vi "Main_control_cRIO.vi"() -> ()   [LabVIEW 2021]
uses:
  <vilib>/platform/TimedLoop/XDataNode/XDataNode.xnode
  <vilib>/Platform/TimedLoop/XDataNode/nitl_modes.ctl
  <vilib>/Platform/TimedLoop/XDataNode/XDNodeRunTimeDep.lvlib
  <vilib>/Platform/TimedLoop/XDataNode/wakeup.ctl
  <vilib>/Platform/TimedLoop/XDataNode/timing_clust.ctl
  <vilib>/rvi/interface/nirviOpenFPGA/nirviOpenFPGA.xnode
  <vilib>/rvi/interface/nirviReadWriteControl/nirviReadWriteControl.xnode
  <vilib>/rvi/interface/nirviCloseFPGA/nirviCloseFPGA.xnode
  SubVIs/DAQ/DAQ_Termopares.lvlib
  SubVIs/CC Modbus/CC_Library.lvlib
  <vilib>/Analysis/NI_AALBase.lvlib
  <vilib>/Analysis/baseanly.llb/Mean (DBL).vi
  <vilib>/Modbus/slave/Modbus Slave.lvclass
  a7aeaaac-04ba-4589-9d9a-9c348744fe2e.vi
  <vilib>/rvi/interface/Simulation/niFpgaSimulationCallBeginRW.vi
  <vilib>/rvi/errors/niLvFpgaAdjustHostInterfaceError.vi
  <vilib>/Modbus/master/Modbus Master.lvclass
  <vilib>/Modbus/slave/Create Slave Instance (TCP).vi
  NiFpgaLv.dll
  <vilib>/Utility/error.llb/Error Cluster From Error Code.vi
  <vilib>/FPGAPlugInAG/Dynamic/niLvFpga_Close_Dynamic.vi
  FPGA Bitfiles/pwmhybrid_FPGATarget_FPGA1_zfi6noby5Tw.lvbitx
  DEV_cRIO Bitron v9_4/FPGA_1.vi
  <vilib>/FPGAPlugInAG/cRIO-9045/niLvFpga_Open_cRIO-9045.vi
  <vilib>/rvi/interface/common/dynamic/niFpgaDynamicAddResources.vi
panel:
  in  "Activar Sim Bitron":bool
  out "LEL":bool
  out "CO":bool
  out "O2":bool
  out "LEL (%)":dbl
  out "CO (%)":dbl
  out "O2 (%)":dbl
  out "Array Warnings":bool[](array[boolean])
  out "Guardando resumen":bool=TRUE
  out "path":path
  out "T estabilidad calor":u32
  out "T transitorio calor":u32
  out "T estabilidad frio":u32
  out "T transitorio frio":u32
  out "Timer 4 (Inicio Estabilidad Calor)":u32
  out "Timer 3 (Inicio Transitorio Calor)":u32
  in  "Configuración":T1(tab)
  in  "Setpoint calor cam":dbl=55.0
  in  "Setpoints peltiers":dbl=85.0
  in  "Setpoint calor corte rampa":dbl=51.0
  in  "Setpoint Frío":dbl=-40.0 min=-28.0 max=70.0 step=0.1
  in  "Setpoint Corte Frío":dbl=-30.0 min=-28.0 max=70.0 step=0.1
  in  "Tiempò en estabilidad de Frío":u32=15
  in  "Tiempo minimo de ciclo":u32=70
  in  "Tiempo maximo de ciclo":u32=90
  in  "Cam ºC/min":dbl=2.2
  in  "Pelt ºC/min":dbl=2.5
  in  "T cliclo (Bitron FSM Sim)":u32
  in  "FSM Bitron Simulacion":i32
  out "DO H2 LAB":bool
  out "Array":dbl[][](array[numeric])
  out "error out":errorcluster
  in  "Test":bool
  in  "Disable PID":bool
  in  "Test PWM":u32[](array[numeric])
  out "PWM array":u32[](array[numeric])
  out "T_valves":dbl[](array[numeric]) format="%0.2f"
  out "PWM 8 (%)":u32
  out "PWM 7 (%)":u32
  out "PWM 6 (%)":u32
  out "PWM 5 (%)":u32
  out "PWM 4 (%)":u32
  out "PWM 3 (%)":u32=50 max=100
  out "SGL values":dbl[](array[numeric])
  out "Int values":u16[](array[numeric])
  out "Guardando en disco":bool
  out "array w/ subset deleted":dbl[][](array[numeric])
  out "Guardar Array":dbl[][](array[numeric])
  out "size(s)":i32
  out "TCP Connection Count":u32
  out "mean_T_valves":dbl format="%0.2f"
  out "Holding registers":u16[](array[numeric])
  out "First Time":bool=TRUE
  out "Timer 1 (Inicio transitorio frio)":u32
  out "Timer 2 (Inicio Estabilidad Frio)":u32
  in  "Rampa_cam":bool
  out "Temp_valves":dbl[](array[numeric]) format="%0.2f"
  in  "Rampa_pelt":bool
  in  "Minutos de medio ciclo":dbl=70.0
  out "Minutos":dbl
  out "Ciclos Totales":dbl
  out "segundos":dbl
  out "días":dbl
  out "Horas":dbl
  out "Minutos Totales":dbl
  out "t ensayo (s)":u64
  in  "Reset tempo":bool
  out "Iteration Duration":i64
  in  "Desconex_Control_Hum":bool
  out "PWM 2 (%)":u32
  out "Program running":bool
  in  "Pausa entrar":bool
  in  "Segmento":u16
  in  "Pausa":bool
  in  "stop Control General":bool
  in  "Run Program":bool
  in  "Entrada digital Bitron":bool
  in  "Cam_Hum_write":dbl min=0.0 max=100.0 step=0.1
  in  "Cam_Write_Set_Hum":bool
  in  "Cam_Temp_write":dbl min=-28.0 max=70.0 step=0.1
  in  "Cam_Write_Set_Temp":bool
  out "Cam_Temp_read":dbl min=-28.0 max=70.0 step=0.1
  out "Cam_Hum_read":dbl min=-28.0 max=70.0 step=0.1
  in  "Setpoint Peltiers":dbl=25.0
  in  "enable_PI":bool
  out "PWM 1 (%)":u32=50 max=100
  in  "STOP ALL":bool
  # "Temporizadores de ciclo"
  # "PWM1TEST"
  # "PWM2TEST"
  # "PWM3TEST"
  # "PWM4TEST"
  # "PWM5TEST"
  # "PWM6TEST"
  # "PWM7TEST"
  # "PWM8TEST"
  # "Peltier_1"
  # "Cámara climática"
  # "min"
  # "min"
  # "min"
  # "min"
  # "segmento"
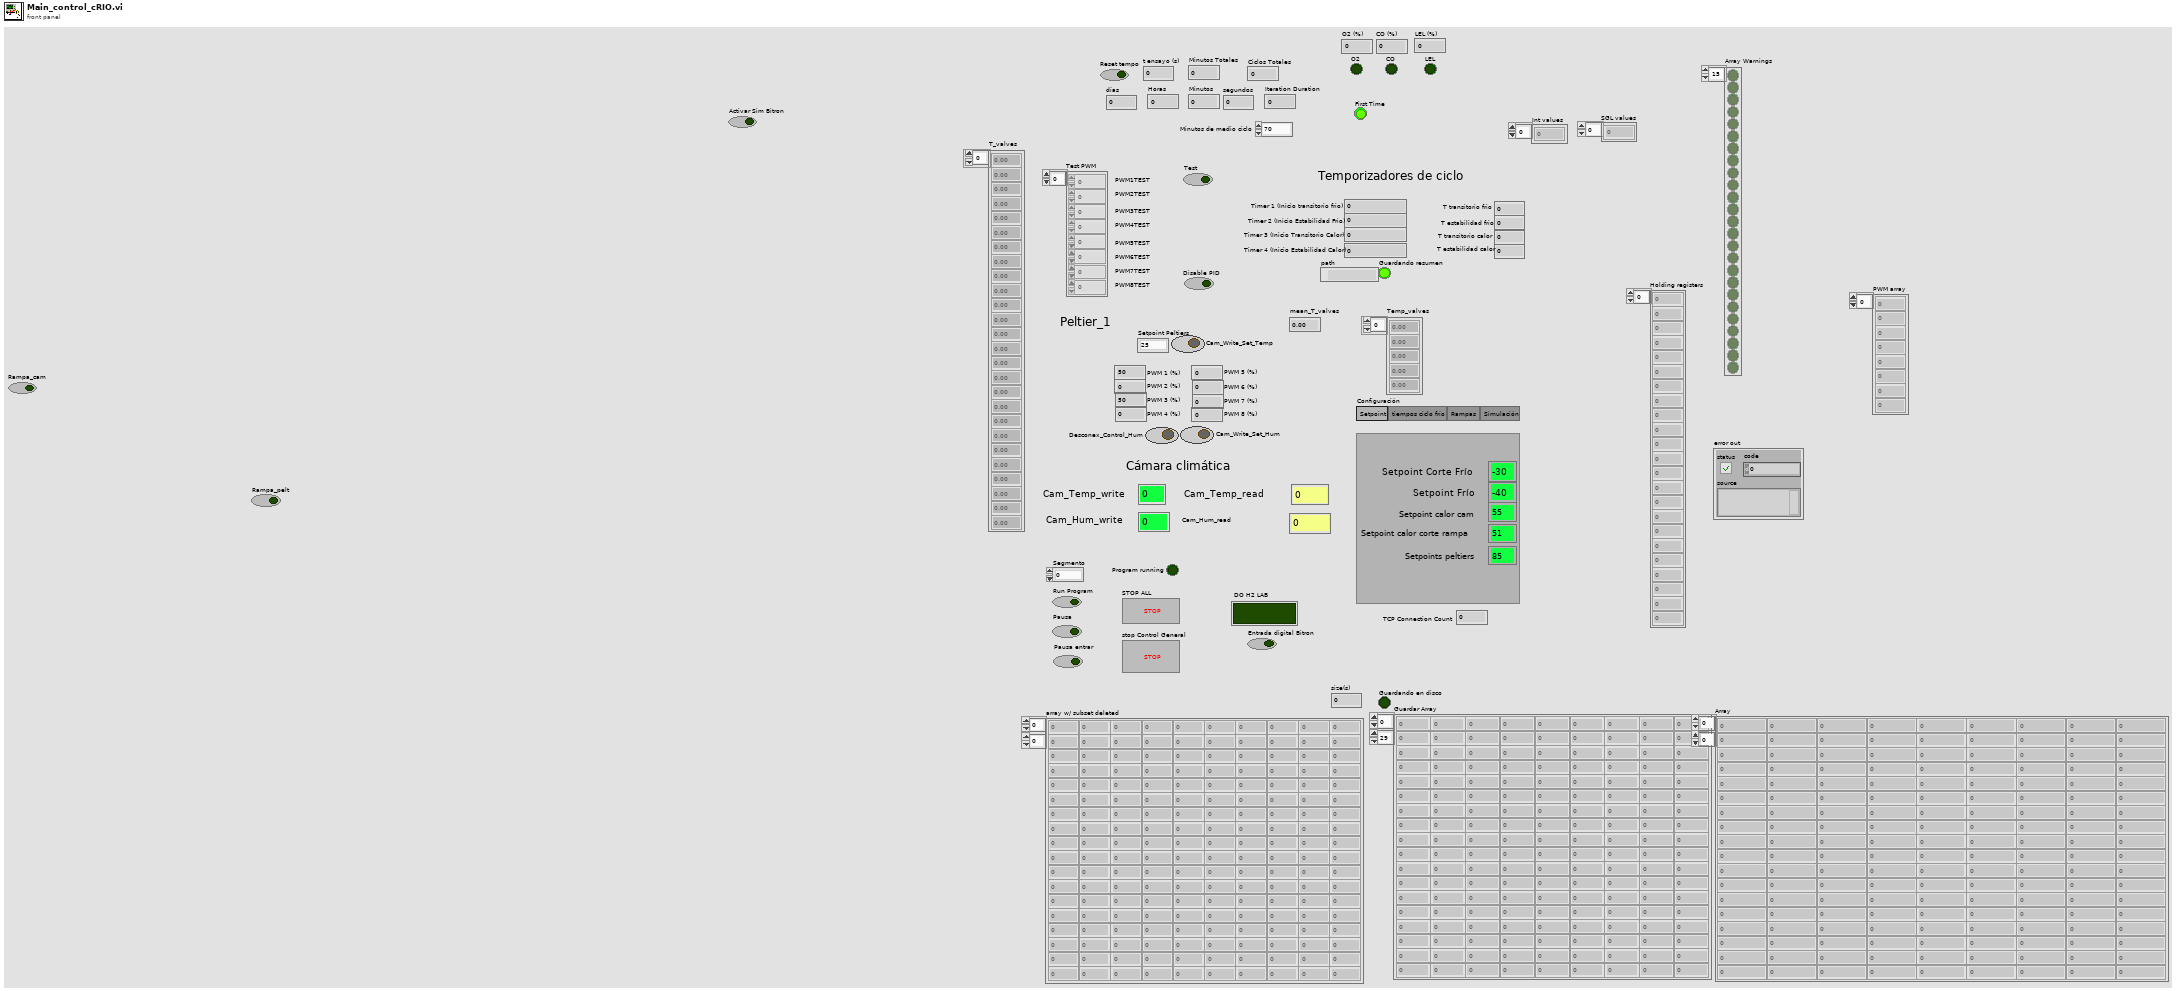
[diagram p1: front panel]
types:
  T1 = enum32{"Setpoint", "tiempos ciclo frío", "Rampas ", "Simulación"}
  T2 = enum8{"Enabled", "Disabled", "Disabled and Grayed Out"}
  T3 = typedef "XDNodeRunTimeDep.lvlib/timing_clust.ctl" = cluster{"Expected End [f-1]":u64, "Actual End [f-1]":u64, "Finished Late? [f-1]":bool, "Expected End [i-1]":u64, "Actual End [i-1]":u64, "Finished Late? [i-1]":bool, "Expected Start [i]":u64, "Actual Start [i]":u64, "Expected Start [f]":u64, "Actual Start [f]":u64, "Source Name":string, "Structure Name":string, "Period":i64, "Deadline":i64, "Offset":i64, "Start":i64, "Priority":i32, "Timeout":i32, "Mode":T4, "Wakeup Reason":T5, "Error":errorcluster, "Source Type":string, "Secondary Source Type":string, "Global End Time":u64, "Global Start Time":u64, "Frame Duration":u64, "Iteration Duration":u64, "Assigned CPU":i32, "I/O Scan Engine Mode":u32}
  T4 = typedef "XDNodeRunTimeDep.lvlib/nitl_modes.ctl" = enum32{"No Change", "Process missed periods, maintain original phase", "Discard missed periods, maintain original phase", "Process missed periods, ignore original phase", "Discard missed periods, ignore original phase"}
  T5 = typedef "XDNodeRunTimeDep.lvlib/wakeup.ctl" = enum32{"Normal", "Aborted", "Asynchronous wakeup", "Timing source error", "Timed loop error", "Timeout"}
  T6 = enum16{"open", "open or create", "create or replace", "create", "open (read-only)"}
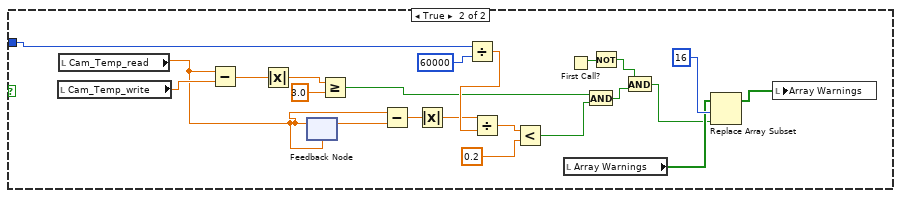
[diagram p3: hidden frame]
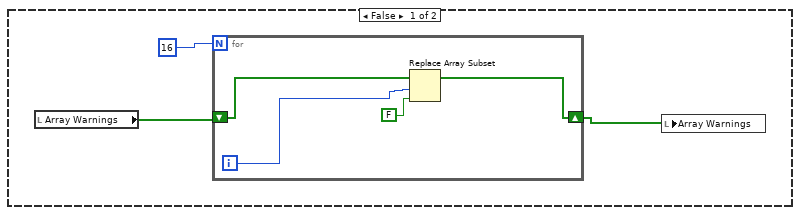
[diagram p4: hidden frame]
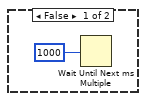
[diagram p7: hidden frame]
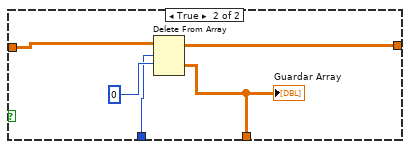
[diagram p8: hidden frame]
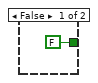
[diagram p9: hidden frame]
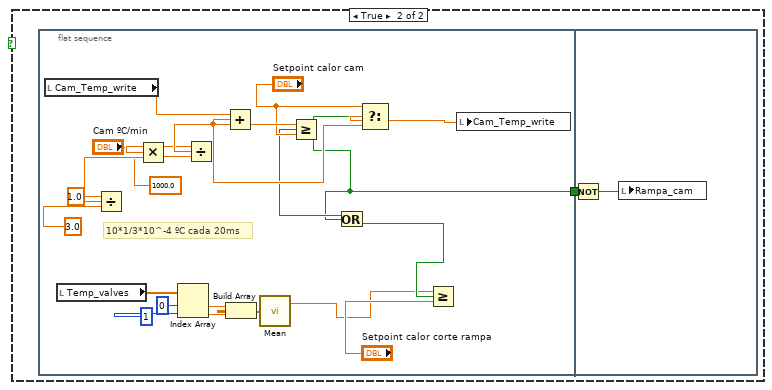
[diagram p12: hidden frame]
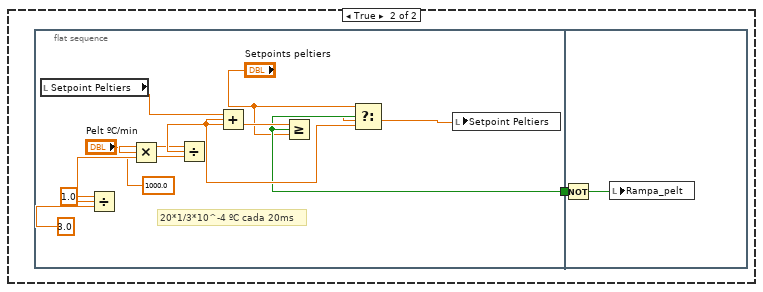
[diagram p13: hidden frame]
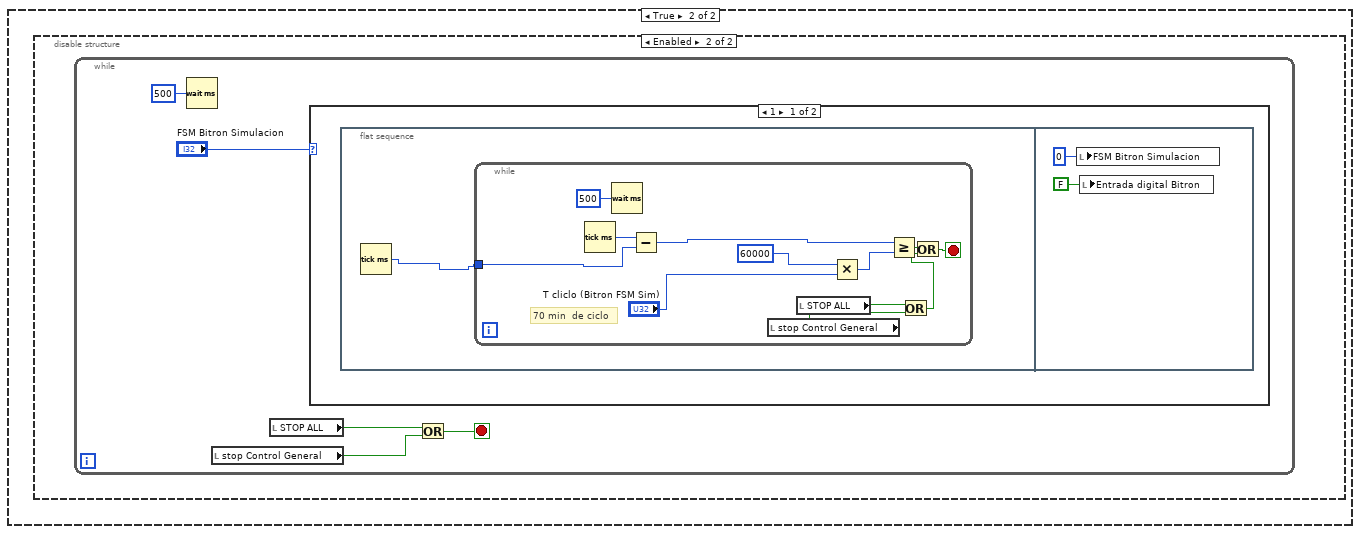
[diagram p14: hidden frame]
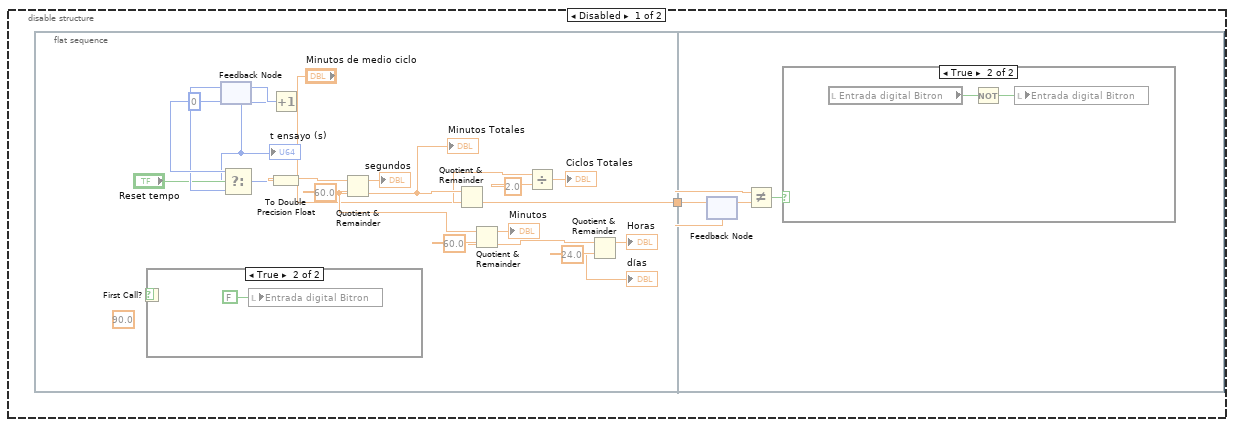
[diagram p15: hidden frame]
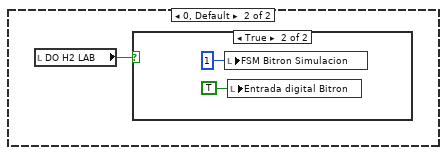
[diagram p18: hidden frame]
diagram:
  n1 = flat-sequence {
    tunnel: [w25] -> w15
    tunnel: [w24] -> w12
    tunnel: [w20] -> w11
    tunnel: [w27] -> w8
    tunnel: [w26] -> w7
    tunnel: [w17] -> w4
    tunnel: [w16] -> w3
    tunnel: w15 -> [w58]
    tunnel: [w57] -> w14
    tunnel: [w56] -> w13
    tunnel: w12 -> [w55]
    tunnel: w11 -> [_]
    tunnel: [w48] -> w10
    tunnel: [w47] -> w9
    tunnel: w8 -> [w44]
    tunnel: w7 -> [w43]
    tunnel: [w42] -> w6
    tunnel: [w41] -> w5
    tunnel: w4 -> [_]
    tunnel: w3 -> [_]
    tunnel: [w29] -> w2
    tunnel: [w30] -> w1
    tunnel: w14 -> [w815]
    tunnel: w13 -> [w814]
    tunnel: w10 -> [w823]
    tunnel: w9 -> [w822]
    tunnel: w6 -> [w818]
    tunnel: w5 -> [w817]
    tunnel: w2 -> [w809]
    tunnel: w1 -> [w810]
    frame #0 {
      w16 = bool[] [FALSE, FALSE, FALSE, FALSE, FALSE, FALSE, FALSE, FALSE, FALSE, FALSE, FALSE, FALSE, FALSE, FALSE, FALSE, FALSE, FALSE, FALSE, FALSE] ("Array Warnings")
      w17 = FALSE ("DO H2 LAB")
      w18 = u32 0 ("PWM 1 (%)")
      w22 = TRUE ("Visible")
      w28 = 10086 items=["J"=10072, "K"=10073, "N"=10077, "R"=10082, "S"=10085, "T"=10086, "B"=10047, "E"=10055] ("thermocouple type")
      w20 = FALSE ("Visible")
      n2 = local write "Entrada digital Bitron"(FALSE ("Entrada digital Bitron")) -> ()
      n3 = call "DAQ_connect.vi"("thermocouple type"=w28, "Array"=tag[] ["Mod2/ai0", "Mod2/ai1", "Mod2/ai2", "Mod2/ai3", "Mod2/ai4", "Mod2/ai5", "Mod2/ai6", "Mod2/ai7", "Mod2/ai8", "Mod2/ai9", "Mod2/ai10", "Mod2/ai11", "Mod2/ai12", "Mod2/ai13", "Mod2/ai14", "Mod2/ai15"]) -> ("error out"=w26:errorcluster, "Refnum out"=w27:refnum<k21>)  [unwired: 8 in]
      "error out" <- w26
      n4 = property on="Cam_Write_Set_Temp" class="Bool (strict)"("Visible"=w22) -> ()  [unwired: 2 in, 2 out]
      n5 = local write "PWM 8 (%)"(w18) -> ()
      n6 = property on="Cam_Write_Set_Hum" class="Bool (strict)"("Visible"=w22) -> ()  [unwired: 2 in, 2 out]
      n7 = local write "PWM 6 (%)"(w18) -> ()
      n8 = local write "PWM 7 (%)"(w18) -> ()
      n9 = local write "PWM 5 (%)"(w18) -> ()
      n10 = local write "PWM 4 (%)"(w18) -> ()
      n11 = local write "PWM 1 (%)"(w18) -> ()
      n12 = local write "PWM 2 (%)"(w18) -> ()
      n13 = local write "Rampa_pelt"(w20) -> ()
      n14 = local write "PWM 3 (%)"(w18) -> ()
      n15 = property on="enable_PI" class="Bool (strict)"("Visible"=w20) -> ()  [unwired: 2 in, 2 out]
      n16 = xnode "Open FPGA VI Reference"() -> ("FPGA VI Reference Out"=w25:refnum<k20>, "error out"=w24:errorcluster)  [unwired: 2 in]
      n17 = property on="Disable PID" class="Bool (strict)"("DisabledEnum"=T2."Disabled" ("Disabled")) -> ()  [unwired: 2 in, 2 out]
      "DO H2 LAB" <- w17
      "Array Warnings" <- w16
    }
    frame #1 {
      # "Running"
      n18 = node-c288() -> (w36:T3)  [unwired: 4 in]
      n19 = node-c288() -> (w60:T3)  [unwired: 4 in]
      n20 = node-c288() -> (w34:T3)  [unwired: 4 in]
      n21 = call "Nanodac_connect.vi"() -> ("error out"=w31:errorcluster, "Modbus Master out"=w32:refnum<class "Modbus Master.lvclass">)  [unwired: 10 in]
      n22 = while "Adquisicion Resumen Datos/ciclo" {
        stop <- w170 stop-if-true
        w171 = FALSE ("Guardando resumen")
        # "CUIDADO! Al volver a empezar el ciclo, el Timer 1 va a ser el del siguiente ciclo, no el del que queremos registrar"
        # "0 -> First Time. Frío hasta -30 y señal bitron\n1 -> Transitorio frio\n2 -> Estabilidad frio\n3 -> Transitorio calor\n4 -> Estabilidad calor"
        # "Datos a guardar por ciclo:\n- Tiempo semiciclo frio\n- Tiempo estabilidad frio\n- Tiempo semiciclo calor\n- Tiempo estabilidad calor"
        n23 = local read "Segmento"() -> (w182:u16)
        n24 = feedback-in #1(w182) -> ()
        n25 = feedback #1(w182) -> (w181:u16)
        n26 = Equal?(x=w182, y=u16 1) -> (x = y?=w179:bool)
        n27 = local read "Program running"() -> (w168:bool)
        n28 = local write "Guardando resumen"(w171) -> ()
        n29 = local read "Segmento"() -> (w173:u16)
        n30 = Not Equal?(x=w181, y=u16 1) -> (x != y?=w178:bool)
        n31 = And(x=w179, y=w178) -> (x .and. y?=w169:bool)
        n32 = And(x=w168, y=w169) -> (x .and. y?=w167:bool)
        n33 = feedback #2(w173) -> (w174:u16)
        n34 = feedback-in #2(w173) -> ()
        n35 = Equal?(x=w173, y=u16 4) -> (x = y?=w176:bool)
        n36 = local read "Program running"() -> (w164:bool)
        n37 = case shown="True" w167 {
          tunnel: w171 -> [_ _]
          frame False {
          }
          frame True {
            n38 = flat-sequence {
              frame #0 {
                n39 = local read "Timer 4 (Inicio Estabilidad Calor)"() -> (w188:u32)
                n40 = local read "Timer 3 (Inicio Transitorio Calor)"() -> (w190:u32)
                n41 = local read "Timer 2 (Inicio Estabilidad Frio)"() -> (w191:u32)
                n42 = local read "Timer 1 (Inicio transitorio frio)"() -> (w189:u32)
                n43 = Subtract(x=w189, y=w188) -> (x-y=→"T estabilidad calor":u32)
                n44 = Subtract(x=w188, y=w190) -> (x-y=→"T transitorio calor":u32)
                n45 = Subtract(x=w190, y=w191) -> (x-y=→"T estabilidad frio":u32)
              }
              frame #1 {
                n46 = while {
                  stop <- w195 stop-if-true
                  n47 = local read "Guardando en disco"() -> (w196:bool)
                  n48 = Not(x=w196) -> (.not. x?=w195:bool)
                  n49 = Wait (ms)(milliseconds to wait=u32 500) -> ()  [unwired: 1 out]
                }
              }
              frame #2 {
                n50 = local read "T estabilidad frio"() -> (w203:u32)
                n51 = local read "T transitorio calor"() -> (w202:u32)
                n52 = local read "path"() -> (w199:path)
                n53 = local read "T transitorio frio"() -> (w204:u32)
                n54 = local read "T estabilidad calor"() -> (w201:u32)
                n55 = TDMS Open(10:T6."open or create" ("operation (0:open)"), 11:w199) -> (0:w209:errorcluster, 3:w210:refnum<k34>)  [unwired: 5 in]
                n56 = Build Array(w204, w203, w202, w201) -> (w200:u32[])
                n57 = TDMS Write(0:w210, 5:"Resumen Ciclos" ("group name in (Untitled)"), 7:string[] ["Time Transitorio frio (s)", "Time estabilidad frio (s)", "Time Transitorio calor (s)", "Time estabilidad calor (s)"] ("channel name(s) in (Untitled)"), 9:w200, 11:w209) -> (4:w208:refnum<k34>, 15:w207:errorcluster)  [unwired: 1 in, 2 out]
                n58 = TDMS Close(8:w207, 11:w208) -> ()  [unwired: 2 out]
                "Guardando resumen" <- TRUE
              }
            }
          }
        }
        n59 = Not Equal?(x=w174, y=u16 4) -> (x != y?=w177:bool)
        n60 = And(x=w176, y=w177) -> (x .and. y?=w166:bool)
        n61 = And(x=w166, y=w164) -> (x .and. y?=w165:bool)
        n62 = case shown="True" w165 {
          frame False {
          }
          frame True {
            n63 = local read "Timer 1 (Inicio transitorio frio)"() -> (w185:u32)
            n64 = local read "Timer 2 (Inicio Estabilidad Frio)"() -> (w184:u32)
            n65 = Subtract(x=w184, y=w185) -> (x-y=→"T transitorio frio":u32)
          }
        }
        n66 = local read "STOP ALL"() -> (w170:bool)
        n67 = Wait (ms)(milliseconds to wait=u32 500) -> ()  [unwired: 1 out]
      }
      n68 = timed-loop "Rampa SP Camara" {
        timing: w36 -> [_]
        timing-out: [_] -> w35
        stop <- w435 stop-if-true
        n69 = node-c288() -> ()  [unwired: 1 in, 1 out]
        n70 = case shown="False" "Rampa_cam" {
          frame False {
            n71 = Wait (ms)(milliseconds to wait=u32 500) -> ()  [unwired: 1 out]
          }
          frame True {
            n72 = flat-sequence {
              tunnel: [w445] -> w437
              tunnel: w437 -> [w460]
              frame #0 {
                # "10*1/3*10^-4 ºC cada 20ms"
                n73 = local read "Cam_Temp_write"() -> (w451:dbl)
                n74 = local read "Temp_valves"() -> (w443:dbl[])
                n75 = Divide(x=1.0, y=3.0) -> (x/y=w457:dbl)
                n76 = Multiply(x="Cam ºC/min", y=w457) -> (x*y=w455:dbl)
                n77 = Index Array(array=w443, index #1=0 ("index"), index #2=1 ("index")) -> (element #1=w440:dbl, element #2=w439:dbl)
                n78 = Divide(x=w455, y=1000.0) -> (x/y=w456:dbl)
                n79 = Add(x=w451, y=w456) -> (x+y=w453:dbl)
                n80 = Build Array(w440, w439) -> (w438:dbl[])
                n81 = call-poly <vilib>:"Mean.vi"("X"=w438) -> ("mean"=w444:dbl)  [unwired: 1 out]
                n82 = Greater Or Equal?(x=w453, y="Setpoint calor cam") -> (x >= y?=w446:bool)
                n83 = Greater Or Equal?(x=w444, y="Setpoint calor corte rampa") -> (x >= y?=w447:bool)
                n84 = Or(x=w446, y=w447) -> (x .or. y?=w445:bool)
                n85 = Select(t="Setpoint calor cam", s=w445, f=w453) -> (s? t:f=w452:dbl)
                n86 = local write "Cam_Temp_write"(w452) -> ()
              }
              frame #1 {
                n87 = Not(x=w460) -> (.not. x?=w461:bool)
                n88 = local write "Rampa_cam"(w461) -> ()
              }
            }
          }
        }
        n89 = local read "STOP ALL"() -> (w435:bool)
        n90 = node-c288() -> ()  [unwired: 1 in, 1 out]
      }
      n91 = timed-loop "FPGA Aquisicion y control" {
        timing: w60 -> [_]
        timing-out: [_] -> w59
        tunnel: w58 -> [w802]
        tunnel: [w801] -> w57
        tunnel: [w800] -> w56
        tunnel: w55 -> [w799]
        tunnel: w44 -> [w798]
        tunnel: w43 -> [w797]
        tunnel: [w796] -> w42
        tunnel: [w795] -> w41
        stop <- "STOP ALL" stop-if-true
        # "1 y 1 de momento, cuando haya mas valvulas, 2 y 2"
        n92 = node-c288() -> ()  [unwired: 1 in, 1 out]
        n93 = local read "PWM 8 (%)"() -> (w779:u32)
        n94 = local read "PWM 6 (%)"() -> (w781:u32)
        n95 = local read "PWM 7 (%)"() -> (w780:u32)
        n96 = local read "PWM 5 (%)"() -> (w782:u32)
        n97 = local read "PWM 4 (%)"() -> (w783:u32)
        n98 = local read "PWM 1 (%)"() -> (w786:u32)
        n99 = local read "PWM 2 (%)"() -> (w785:u32)
        n100 = local read "PWM 3 (%)"() -> (w784:u32)
        n101 = xnode "Read/Write Control"("FPGA VI Reference In"=w802, "error in"=w799) -> ("FPGA VI Reference Out"=w801:refnum<k20>, "error out"=w800:errorcluster)  [unwired: 8 in]
        n102 = call "DAQ_read_T_dT.vi"("error in (no error)"=w797, "Refnum in"=w798) -> ("error out"=w795:errorcluster, "data"=w794:dbl[], "Refnum out"=w796:refnum<k21>)  [unwired: 7 in]
        "Temp_valves" <- w794
        "T_valves" <- w794
        n103 = Build Array(w786, w785, w784, w783, w782, w781, w780, w779) -> (→"PWM array":u32[])
        n104 = call "Sort 1D Array.vim"("unsorted array"=w794) -> ("sorted array"=w790:dbl[])  [unwired: 10 in]
        n105 = Array Size(array=w790) -> (size(s)=w792:i32)
        n106 = Subtract(x=w792, y=1) -> (x-y=w793:i32)
        n107 = Array Subset(array=w790, index=1, length=w793) -> (w788:dbl[])
        n108 = call-poly <vilib>:"Mean.vi"("X"=w788) -> ("mean"=→"mean_T_valves":dbl)  [unwired: 1 out]
        n109 = node-c288() -> ()  [unwired: 1 in, 1 out]
      }
      n110 = timed-loop "Warnings/Errores" {
        timing: w34 -> [_]
        timing-out: [_] -> w33
        stop <- w74 stop-if-true
        n111 = node-c288() -> ()  [unwired: 1 in, 1 out]
        n112 = local read "Program running"() -> (w77:bool)
        n113 = local read "Pausa"() -> (w78:bool)
        n114 = Not(x=w78) -> (.not. x?=w76:bool)
        n115 = And(x=w77, y=w76) -> (x .and. y?=w75:bool)
        n116 = case shown="True" w75 {
          frame False {
          }
          frame True {
            # "0 -> First Time. Frío hasta -30 y señal bitron\n1 -> Transitorio frio\n2 -> Estabilidad frio\n3 -> Transitorio calor\n4 -> Estabilidad calor"
            # "Si estamos en semiciclo de calor\ny no hay pausa"
            n117 = local read "Segmento"() -> (w110:u16)
            n118 = Tick Count (ms)() -> (millisecond timer value=w104:u32)
            n119 = local read "LEL (%)"() -> (w96:dbl)
            n120 = feedback-in #3(w104) -> ()
            n121 = feedback #3(w104) -> (w103:u32)
            n122 = local read "Array Warnings"() -> (w92:bool[])
            n123 = Equal?(x=w110, y=u16 3) -> (x = y?=w107:bool)
            n124 = Equal?(x=w110, y=u16 4) -> (x = y?=w106:bool)
            n125 = Subtract(x=w104, y=w103) -> (x-y=w101:u32)
            n126 = Greater?(x=w96, y=3.0) -> (0:w90:bool)
            n127 = Or(x=w107, y=w106) -> (x .or. y?=w105:bool)
            n128 = Replace Array Subset(array=w92, new element=w90, index=17) -> (w89:bool[])
            n129 = Greater Or Equal?(x=w101, y=u32 1000) -> (x >= y?=w100:bool)
            n130 = Array Subset(array=w89, index=0, length=19) -> (w82:bool[])
            n131 = case shown="True" w105 {
              frame False {
                n132 = local read "Array Warnings"() -> (w138:bool[])
                n133 = for {
                  N: 16 -> [_]
                  shift-right: [w140] -> w137
                  shift-left: w138 -> [w141]
                  i -> [w143]
                  n134 = Replace Array Subset(array=w141, new element=FALSE ("new element/subarray"), index=w143) -> (w140:bool[])
                }
                n135 = local write "Array Warnings"(w137) -> ()
              }
              frame True {
                n136 = local read "Array Warnings"() -> (w145:bool[])
                n137 = local read "Setpoint Peltiers"() -> (w148:dbl)
                n138 = local read "T_valves"() -> (w147:dbl[])
                n139 = for {
                  N: 16 -> [_]
                  tunnel: w148 -> [w155]
                  tunnel: w147 -> [w153]
                  shift-right: [w149] -> w144
                  shift-left: w145 -> [w150]
                  i -> [w152]
                  n140 = Index Array(array=w153, index=w152) -> (element=w151:dbl)
                  n141 = Subtract(x=w155, y=w151) -> (x-y=w158:dbl)
                  n142 = Absolute Value(x=w158) -> (abs(x)=w157:dbl)
                  n143 = Greater?(x=w157, y=20.0) -> (0:w154:bool)
                  n144 = Replace Array Subset(array=w150, new element=w154, index=w152) -> (w149:bool[])
                }
                n145 = local write "Array Warnings"(w144) -> ()
              }
            }
            n146 = case shown="False" w100 {
              tunnel: w101 -> [_ w132]
              frame False {
                n147 = local read "Array Warnings"() -> (w114:bool[])
                n148 = Replace Array Subset(array=w114, new element=FALSE ("new element/subarray"), index=16) -> (w111:bool[])
                n149 = local write "Array Warnings"(w111) -> ()
              }
              frame True {
                n150 = local read "Cam_Temp_write"() -> (w121:dbl)
                n151 = local read "Cam_Temp_read"() -> (w119:dbl)
                n152 = Subtract(x=w119, y=w121) -> (x-y=w136:dbl)
                n153 = Absolute Value(x=w136) -> (abs(x)=w135:dbl)
                n154 = feedback #4(w119) -> (w120:dbl)
                n155 = feedback-in #4(w119) -> ()
                n156 = Greater Or Equal?(x=w135, y=3.0) -> (x >= y?=w126:bool)
                n157 = Subtract(x=w119, y=w120) -> (x-y=w133:dbl)
                n158 = Absolute Value(x=w133) -> (abs(x)=w129:dbl)
                n159 = Divide(x=w132, y=u32 60000) -> (x/y=w130:dbl)
                n160 = Divide(x=w129, y=w130) -> (x/y=w128:dbl)
                n161 = Less?(x=w128, y=0.2) -> (x < y?=w125:bool)
                n162 = local read "Array Warnings"() -> (w116:bool[])
                n163 = First Call?() -> (First Call?: T/F=w122:bool)
                n164 = And(x=w126, y=w125) -> (x .and. y?=w124:bool)
                n165 = Not(x=w122) -> (.not. x?=w123:bool)
                n166 = And(x=w123, y=w124) -> (x .and. y?=w115:bool)
                n167 = Replace Array Subset(array=w116, new element=w115, index=16) -> (w118:bool[])
                n168 = local write "Array Warnings"(w118) -> ()
              }
            }
            n169 = local write "Array Warnings"(w82) -> ()
            n170 = local read "O2 (%)"() -> (w81:dbl)
            n171 = local read "Array Warnings"() -> (w95:bool[])
            n172 = Greater?(x=w81, y=25.0) -> (0:w97:bool)
            n173 = Less?(x=w81, y=10.0) -> (x < y?=w79:bool)
            n174 = Or(x=w97, y=w79) -> (x .or. y?=w93:bool)
            n175 = Replace Array Subset(array=w95, new element=w93, index=18) -> (w84:bool[])
            n176 = Array Subset(array=w84, index=0, length=19) -> (w83:bool[])
            n177 = local write "Array Warnings"(w83) -> ()
          }
        }
        n178 = local read "STOP ALL"() -> (w74:bool)
        n179 = node-c288() -> ()  [unwired: 1 in, 1 out]
      }
      n180 = while "MODBUS CC NANODAC" {
        tunnel: w32 -> [w73]
        tunnel: w31 -> [w72]
        tunnel: [w62] -> w30
        tunnel: [w61] -> w29
        stop <- w71 stop-if-true
        n181 = call "Nanodac_lectura.vi"("Modbus Master in"=w73, "error in (no error)"=w72) -> ("Modbus Master out"=w62:refnum<class "Modbus Master.lvclass">, 16:"O2, CO, LEL"=w69:dbl[], 17:"O2, CO, LEL"=w70:bool[], "error out"=w61:errorcluster)  [unwired: 14 in]
        n182 = Index Array(array=w70) -> (element #1=→"O2":bool, element #2=→"CO":bool, element #3=→"LEL":bool)  [unwired: 3 in]
        n183 = Index Array(array=w69) -> (element #1=→"O2 (%)":dbl, element #2=→"CO (%)":dbl, element #3=→"LEL (%)":dbl)  [unwired: 3 in]
        n184 = local read "STOP ALL"() -> (w71:bool)
      }
      n185 = node-c288(w35) -> ()  [unwired: 1 out]
      n186 = node-c288() -> (w38:T3)  [unwired: 4 in]
      n187 = timed-loop "Rampa SP Peltiers" {
        timing: w38 -> [_]
        timing-out: [_] -> w37
        stop <- w467 stop-if-true
        n188 = node-c288() -> ()  [unwired: 1 in, 1 out]
        n189 = case shown="False" "Rampa_pelt" {
          frame False {
            n190 = Wait (ms)(milliseconds to wait=u32 500) -> ()  [unwired: 1 out]
          }
          frame True {
            n191 = flat-sequence {
              tunnel: [w474] -> w469
              tunnel: w469 -> [w482]
              frame #0 {
                # "20*1/3*10^-4 ºC cada 20ms"
                n192 = local read "Setpoint Peltiers"() -> (w472:dbl)
                n193 = Divide(x=1.0, y=3.0) -> (x/y=w479:dbl)
                n194 = Multiply(x="Pelt ºC/min", y=w479) -> (x*y=w477:dbl)
                n195 = Divide(x=w477, y=1000.0) -> (x/y=w478:dbl)
                n196 = Add(x=w472, y=w478) -> (x+y=w475:dbl)
                n197 = Greater Or Equal?(x=w475, y="Setpoints peltiers") -> (x >= y?=w474:bool)
                n198 = Select(t="Setpoints peltiers", s=w474, f=w475) -> (s? t:f=w473:dbl)
                n199 = local write "Setpoint Peltiers"(w473) -> ()
              }
              frame #1 {
                n200 = Not(x=w482) -> (.not. x?=w483:bool)
                n201 = local write "Rampa_pelt"(w483) -> ()
              }
            }
          }
        }
        n202 = local read "STOP ALL"() -> (w467:bool)
        n203 = node-c288() -> ()  [unwired: 1 in, 1 out]
      }
      n204 = node-c288(w59) -> ()  [unwired: 1 out]
      n205 = while "Guardado de Datos" {
        stop <- w212 stop-if-true
        n206 = local read "Program running"() -> (w211:bool)
        n207 = case shown="True" w211 {
          frame False {
            n208 = Wait Until Next ms Multiple(millisecond multiple=u32 1000 ("milliseconds to wait")) -> ()  [unwired: 1 out]
          }
          frame True {
            w222 = dbl[][] []
            n209 = Get Date/Time In Seconds() -> (seconds since 1Jan1904=w221:timestamp)
            n210 = Format Date/Time String(time format string (%c)="%Y_%m_%d_%H_%M", seconds (now)=w221) -> (date/time string=w217:string)  [unwired: 1 in]
            n211 = local write "array w/ subset deleted"(w222) -> ()
            n212 = local write "Guardar Array"(w222) -> ()
            n213 = Concatenate Strings("/media/sdb1/Datos_Bitron/" ("string"), w217, "_data CC.tdms" ("string")) -> (w218:string)
            n214 = String To Path(string=w218) -> (path=w215:path)
            "path" <- w215
            n215 = while {
              shift-right: [w272] -> _
              shift-left: w222 -> [w275]
              tunnel: w215 -> [w263]
              tunnel: [FALSE ("stop Control General")] -> w214
              i -> [w280]
              stop <- w246 stop-if-true
              # "10 minutos = 599"
              n216 = local read "Program running"() -> (w240:bool)
              n217 = local read "enable_PI"() -> (w239:bool)
              n218 = local read "Entrada digital Bitron"() -> (w238:bool)
              n219 = local read "Run Program"() -> (w237:bool)
              n220 = local read "Pausa"() -> (w236:bool)
              n221 = local read "Pausa entrar"() -> (w235:bool)
              n222 = local read "stop Control General"() -> (w234:bool)
              n223 = local read "DO H2 LAB"() -> (w231:bool)
              n224 = local read "TCP Connection Count"() -> (w252:u32)
              n225 = local read "SGL values"() -> (w261:dbl[])
              n226 = local read "Int values"() -> (w262:u16[])
              n227 = local read "Array Warnings"() -> (w225:bool[])
              n228 = Tick Count (ms)() -> (millisecond timer value=w266:u32)
              n229 = To Double Precision Float(number=w262) -> (double precision float=w260:dbl[])
              n230 = To Double Precision Float(number=w261) -> (double precision float=w259:dbl[])
              n231 = Divide(x=w266, y=u32 1000) -> (x/y=w258:dbl)
              n232 = Greater?(x=w252, y=u32 0) -> (0:w250:bool)
              n233 = Boolean To (0,1)(Boolean=w250) -> (0, 1=w254:i16)
              n234 = To Double Precision Float(number=w254) -> (double precision float=w253:dbl)
              n235 = Build Array(w240, w239, w238, w237, w236, w235, w234, w231) -> (w233:bool[])
              n236 = Boolean To (0,1)(Boolean=w225) -> (0, 1=w226:i16[])
              n237 = Build Array(w253) -> (w232:dbl[])
              n238 = Boolean To (0,1)(Boolean=w233) -> (0, 1=w256:i16[])
              n239 = To Double Precision Float(number=w226) -> (double precision float=w224:dbl[])
              n240 = Build Array(w258) -> (w257:dbl[])
              n241 = To Double Precision Float(number=w256) -> (double precision float=w255:dbl[])
              n242 = Transpose 2D Array(2D array=w275) -> (transposed array=w274:dbl[][])
              n243 = Build Array (concatenate)(w257, w260, w259, w255, w232, w224) -> (w281:dbl[])
              n244 = Insert Into Array(array=w274, new element=w281) -> (w277:dbl[][])  [unwired: 2 in]
              n245 = Transpose 2D Array(2D array=w277) -> (transposed array=w271:dbl[][])
              n246 = Array Size(array=w271) -> (size(s)=w270:i32[])
              n247 = Index Array(array=w270, index=1) -> (element=w269:i32)
              "size(s)" <- w269
              n248 = local read "stop Control General"() -> (w244:bool)
              n249 = local read "Program running"() -> (w248:bool)
              n250 = Quotient & Remainder(x=w280, y=599) -> (floor(x/y)=w276:i32)  [unwired: 1 out]
              n251 = local read "STOP ALL"() -> (w245:bool)
              n252 = local read "Guardando resumen"() -> (w230:bool)
              n253 = feedback-in #5(w276) -> ()
              n254 = feedback #5(w276) -> (w278:i32)
              n255 = Not Equal?(x=w276, y=w278) -> (x != y?=w249:bool)
              n256 = And(x=w249, y=w248) -> (x .and. y?=w229:bool)
              n257 = Or(x=w245, y=w244) -> (x .or. y?=w243:bool)
              n258 = Not(x=w230) -> (.not. x?=w228:bool)
              n259 = And(x=w228, y=w229) -> (x .and. y?=w227:bool)
              n260 = Or(x=w227, y=w243) -> (x .or. y?=w247:bool)
              "Guardando en disco" <- w247
              n261 = case shown="False" w247 {
                tunnel: w277 -> [w283 w286]
                tunnel: [w283 w288] -> w273
                tunnel: w269 -> [_ w285]
                tunnel: [dbl[][] [] w284] -> w241
                frame False {
                }
                frame True {
                  n262 = Delete From Array(array=w286, length=w285, index (row)=0) -> (deleted portion=w284:dbl[][], array with subset deleted=w288:dbl[][])  [unwired: 1 in]
                  "Guardar Array" <- w284
                }
              }
              "array w/ subset deleted" <- w273
              n263 = Transpose 2D Array(2D array=w241) -> (transposed array=w267:dbl[][])
              n264 = case shown="True" w247 {
                tunnel: string[] ["Time", "Segmento", "PWM1 (%)", "PWM2 (%)", "PWM3 (%)", "PWM4 (%)", "PWM5 (%)", "PWM6 (%)", "PWM7 (%)", "PWM8 (%)", "Setpoint T Peltier (ºC)", "T Valve 1 (ºC)", "T Valve 2 (ºC)", "T Valve 3 (ºC)", "T Valve 4 (ºC)", "T Valve 5 (ºC)", "T Valve 6 (ºC)", "T Valve 7 (ºC)", "T Valve 8 (ºC)", "Tª Bob V1 (ºC)", "Tª Bob V2 (ºC)", "Tª Bob V3 (ºC)", "Tª Bob V4 (ºC)", "Tª Bob V5 (ºC)", "Tª Bob V6 (ºC)", "Tª Bob V7 (ºC)", "Tª Bob V8 (ºC)", "HR RD CC (%)", "SP HR WR CC (%)", "T RD CC (ºC)", "SP T WR CC (ºC)", "Program Status", "Enable PI", "Entrada Bitron", "Run Program", "Pause", "Pause Entrar", "Stop control general", "DO H2 Lab", "Comunicación con PC", "W1.1", "W1.2", "W1.3", "W1.4", "W1.5", "W1.6", "W1.7", "W1.8", "W1.9", "W1.10", "W1.11", "W1.12", "W1.13", "W1.14", "W1.15", "W1.16", "W2", "W3", "W4"] -> [_ w294]
                tunnel: w267 -> [_ w293]
                tunnel: w263 -> [_ w292]
                tunnel: w243 -> [_ w291]
                tunnel: [FALSE ("STOP ALL") w290] -> w246
                frame False {
                }
                frame True {
                  n265 = flat-sequence {
                    tunnel: w294 -> [w300]
                    tunnel: w293 -> [w297]
                    tunnel: w292 -> [w296]
                    tunnel: w291 -> [w295]
                    tunnel: [w295] -> w290
                    frame #0 {
                      n266 = disable-structure shown="Disabled" {
                        frame Disabled {
                          n267 = call <vilib>:"Application Directory.vi"() -> ("Application Directory"=w306:path)
                          n268 = Build Path(base path=w306) -> (appended path=w305:path)  [unwired: 1 in]
                          n269 = Build Path(base path=w305, name or relative path=path "data CC.tdms") -> ()  [unwired: 1 out]
                        }
                        frame Enabled {
                        }
                      }
                      n270 = TDMS Open(10:T6."open or create" ("operation (0:open)"), 11:w296) -> (0:w302:errorcluster, 3:w303:refnum<k34>)  [unwired: 5 in]
                      n271 = TDMS Write(0:w303, 5:"Cámara climática" ("group name in (Untitled)"), 7:w300, 9:w297, 11:w302) -> (4:w299:refnum<k34>, 15:w298:errorcluster)  [unwired: 1 in, 2 out]
                      n272 = TDMS Close(8:w298, 11:w299) -> ()  [unwired: 2 out]
                      "Array" <- w297
                    }
                  }
                }
              }
              n273 = Transpose 2D Array(2D array=w273) -> (transposed array=w272:dbl[][])
              n274 = Wait Until Next ms Multiple(millisecond multiple=u32 10000 ("milliseconds to wait")) -> ()  [unwired: 1 out]
            }
            n275 = local write "stop Control General"(w214) -> ()
          }
        }
        n276 = local read "STOP ALL"() -> (w212:bool)
      }
      n277 = while "Modbus Slave" {
        stop <- w308 stop-if-true
        n278 = call-poly <vilib>:"Create Slave Instance.vi"() -> ("error out"=w311:errorcluster, "TCP slave instance"=w312:refnum<class "Modbus Slave.lvclass">)  [unwired: 10 in]
        n279 = while {
          shift-right: [w324] -> w310
          shift-left: w312 -> [w326]
          shift-right: [w323] -> w309
          shift-left: w311 -> [w325]
          stop <- w318 stop-if-true
          n280 = property class="Modbus Slave"(reference=w326, error in=w325) -> (reference out=w324:refnum<class "Modbus Slave.lvclass">, error out=w323:errorcluster, "Data Access:TCP Connection Count"=w322:u32)
          "TCP Connection Count" <- w322
          n281 = Not Equal?(x=w322, y=u32 0) -> (x != y?=w320:bool)
          n282 = local read "STOP ALL"() -> (w319:bool)
          n283 = Or(x=w320, y=w319) -> (x .or. y?=w318:bool)
        }
        n284 = node-c288() -> (w317:T3)  [unwired: 4 in]
        n285 = timed-loop {
          timing: w317 -> [_]
          timing-out: [_] -> w316
          shift-right: [w363] -> w314
          shift-left: w310 -> [w374]
          shift-right: [w362] -> w313
          shift-left: w309 -> [w372]
          shift-right: [w365] -> _
          shift-left: u16[] [0, 0, 0, 0, 0, 0, 0, 0, 0, 0, 0, 0, 0, 0, 0, 0, 0, 0, 0, 0, 0, 0, 0, 0, 0, 0, 0, 0, 0, 0, 0, 0, 0, 0, 0, 0, 0, 0, 0, 0, 0, 0, 0] -> [w366]
          stop <- w358 stop-if-true
          # "Temp_BobV3-8"
          # "Temp_valves\nTemp_bobs"
          n286 = node-c288() -> ()  [unwired: 1 in, 1 out]
          n287 = local read "Entrada digital Bitron"() -> (w347:bool)
          n288 = local read "Array Warnings"() -> (w327:bool[])
          n289 = local read "Program running"() -> (w379:bool)
          n290 = local read "DO H2 LAB"() -> (w334:bool)
          n291 = local read "T_valves"() -> (w342:dbl[])
          n292 = local read "enable_PI"() -> (w378:bool)
          n293 = local read "Cam_Temp_write"() -> (w343:dbl)
          n294 = local read "Cam_Temp_read"() -> (w344:dbl)
          n295 = local read "Cam_Hum_read"() -> (w346:dbl)
          n296 = local read "Cam_Hum_write"() -> (w345:dbl)
          n297 = local read "Setpoint Peltiers"() -> (w377:dbl)
          n298 = Build Array (concatenate)(w379, w378, w347, w334, w327) -> (w373:bool[])
          n299 = Build Array(w346, w345, w344, w343) -> (w340:dbl[])
          n300 = Build Array(w377) -> (w341:dbl[])
          n301 = local read "PWM array"() -> (w336:u32[])
          n302 = local read "Segmento"() -> (w376:u16)
          n303 = Build Array (concatenate)(w341, w342, w340) -> (w339:dbl[])
          "SGL values" <- w339
          n304 = Array Size(array=w339) -> (size(s)=w367:i32)
          n305 = To Unsigned Word Integer(number=w336) -> (unsigned 16bit integer=w337:u16[])
          n306 = call-dynamic "Write Multiple Coils.vi"("error in (no error)"=w372, "coil values"=w373, "starting address"=u16 1, "Modbus slave in"=w374) -> ("error out"=w369:errorcluster, "Modbus slave out"=w370:refnum<class "Modbus Slave.lvclass">)  [unwired: 6 in]
          n307 = Build Array(w376) -> (w338:u16[])
          n308 = Build Array (concatenate)(w338, w337) -> (w335:u16[])
          "Int values" <- w335
          n309 = for {
            N: w367 -> [_]
            tunnel: w339 -> [w429] mode=indexing
            shift-right: [w420] -> w365
            shift-left: w366 -> [w421]
            i -> [w428]
            n310 = call "double_2u16.vi"("Entrada"=w429) -> ("Salida 2"=w425:u16, "Salida 1"=w426:u16)  [unwired: 9 in]
            n311 = Multiply(x=2, y=w428) -> (x*y=w424:i32)
            n312 = Add(x=1, y=w424) -> (x+y=w422:i32)
            n313 = Replace Array Subset(array=w421, new element #1=w426, index #1=w424, new element #2=w425, index #2=w422) -> (w420:u16[])
          }
          n314 = for {
            tunnel: w335 -> [w419] mode=indexing
            tunnel: [w417] -> w364 mode=indexing
            n315 = Add(x=w419, y=u16 10000) -> (x+y=w417:u16)
          }
          n316 = Build Array (concatenate)(w364, w365) -> (w368:u16[])
          "Holding registers" <- w368
          n317 = call-dynamic "Write Multiple Holding Registers.vi"("error in (no error)"=w369, "holding register values"=w368, "starting address"=u16 100, "Modbus slave in"=w370) -> ("error out"=w355:errorcluster, "Modbus slave out"=w356:refnum<class "Modbus Slave.lvclass">)  [unwired: 6 in]
          n318 = call-dynamic "Read Coils.vi"("error in (no error)"=w355, "number of coils"=u16 6, "starting address"=u16 200, "Modbus slave in"=w356) -> ("error out"=w331:errorcluster, "coil values"=w349:bool[], "Modbus slave out"=w332:refnum<class "Modbus Slave.lvclass">)  [unwired: 5 in]
          n319 = Index Array(array=w349) -> (element #1=w352:bool, element #2=w351:bool, element #3=w350:bool, element #4=w348:bool, element #5=w329:bool, element #6=w328:bool)  [unwired: 6 in]
          n320 = local write "Run Program"(w352) -> ()
          n321 = local write "Pausa"(w351) -> ()
          n322 = local write "Pausa entrar"(w350) -> ()
          n323 = local write "stop Control General"(w348) -> ()
          n324 = local write "Activar Sim Bitron"(w328) -> ()
          n325 = case shown="True" w329 {
            tunnel: [w381 w398] -> w333
            tunnel: w332 -> [w381 w400]
            tunnel: w331 -> [w380 w399]
            tunnel: [w380 w397] -> w330
            frame False {
            }
            frame True {
              w384 = u16 22 ("number of holding registers")
              n326 = Quotient & Remainder(x=w384, y=u16 2) -> (floor(x/y)=w382:u16)  [unwired: 1 out]
              n327 = call-dynamic "Read Holding Registers.vi"("error in (no error)"=w399, "number of holding registers"=w384, "starting address"=u16 300, "Modbus slave in"=w400) -> ("error out"=w397:errorcluster, "register values"=w401:u16[], "Modbus slave out"=w398:refnum<class "Modbus Slave.lvclass">)  [unwired: 5 in]
              n328 = for {
                N: w382 -> [_]
                tunnel: [w409] -> w396 mode=indexing
                tunnel: w401 -> [w405]
                i -> [w416]
                n329 = Multiply(x=2, y=w416) -> (x*y=w414:i32)
                n330 = Add(x=w414, y=1) -> (x+y=w412:i32)
                n331 = Index Array(array=w405, index #1=w414, index #2=w412) -> (element #1=w404:u16, element #2=w403:u16)
                n332 = Join Numbers(hi=w404, lo=w403) -> ((hi.lo)=w411:u32)
                n333 = To Single Precision Float(number=w411) -> (single precision float=w408:sgl)
                n334 = Subtract(x=w408, y=sgl 10000.0) -> (x-y=w406:sgl)
                n335 = Divide(x=w406, y=sgl 100.0) -> (x/y=w409:sgl)
              }
              n336 = Index Array(array=w396) -> (element #1=w395:sgl, element #2=w394:sgl, element #3=w393:sgl, element #4=w392:sgl, element #5=w391:sgl, element #6=w390:sgl, element #7=w389:sgl, element #8=w388:sgl, element #9=w387:sgl, element #10=w386:sgl, element #11=w385:sgl)  [unwired: 11 in]
              n337 = local write "Tiempò en estabilidad de Frío"(w390) -> ()
              n338 = local write "Setpoint calor corte rampa"(w392) -> ()
              n339 = local write "Tiempo maximo de ciclo"(w388) -> ()
              n340 = local write "Tiempo minimo de ciclo"(w389) -> ()
              n341 = local write "T cliclo (Bitron FSM Sim)"(w385) -> ()
              n342 = local write "Setpoint Corte Frío"(w395) -> ()
              n343 = local write "Setpoint calor cam"(w393) -> ()
              n344 = local write "Setpoints peltiers"(w391) -> ()
              n345 = local write "Setpoint Frío"(w394) -> ()
              n346 = local write "Cam ºC/min"(w387) -> ()
              n347 = local write "Pelt ºC/min"(w386) -> ()
            }
          }
          n348 = property class="Modbus Slave"(reference=w333, error in=w330) -> (reference out=w363:refnum<class "Modbus Slave.lvclass">, error out=w362:errorcluster, "Data Access:TCP Connection Count"=w361:u32)
          n349 = local read "STOP ALL"() -> (w357:bool)
          n350 = Equal?(x=w361, y=u32 0) -> (x = y?=w359:bool)
          n351 = Or(x=w359, y=w357) -> (x .or. y?=w358:bool)
          n352 = node-c288() -> ()  [unwired: 1 in, 1 out]
        }
        n353 = node-c288(w316) -> ()  [unwired: 1 out]
        n354 = local read "STOP ALL"() -> (w308:bool)
        n355 = call-dynamic "Close.vi"("error in (no error)"=w313, "Modbus slave in"=w314) -> ()  [unwired: 9 in, 1 out]
      }
      n356 = node-c288(w33) -> ()  [unwired: 1 out]
      n357 = node-c288(w37) -> ()  [unwired: 1 out]
      n358 = call "Eurotherm_connect.vi"() -> ("error out"=w49:errorcluster, "Modbus Master out"=w50:refnum<class "Modbus Master.lvclass">)  [unwired: 10 in]
      n359 = node-c288() -> (w46:T3)  [unwired: 4 in]
      n360 = node-c288() -> (w40:T3)  [unwired: 4 in]
      n361 = timed-loop "FSM Control" {
        timing: w46 -> [_]
        timing-out: [_] -> w45
        stop <- w550 stop-if-true
        w549 = FALSE ("Pausa")
        w551 = u16 0 ("Segmento_temp")
        # "Reset Variables locales"
        # "Condiciones inicales T ambiente"
        n362 = node-c288() -> ()  [unwired: 1 in, 1 out]
        n363 = local write "Cam_Write_Set_Temp"(TRUE ("Enable_Temp_write")) -> ()
        n364 = local write "Cam_Temp_write"(25.0 ("Setpoint_temp_write")) -> ()
        n365 = local write "DO H2 LAB"(FALSE ("DO H2 LAB")) -> ()
        n366 = local write "Pausa entrar"(w549) -> ()
        n367 = local write "Segmento"(w551) -> ()
        n368 = local write "enable_PI"(w549) -> ()
        n369 = local write "Pausa"(w549) -> ()
        n370 = case shown="True" "Run Program" {
          tunnel: w551 -> [_ _]
          tunnel: w549 -> [_ _]
          frame False {
          }
          frame True {
            # "Main"
            n371 = while {
              tunnel: [FALSE ("Run Program")] -> w555
              stop <- w557 stop-if-true
              # "0 -> First Time. Frío hasta -30 y señal bitron\n1 -> Transitorio frio\n2 -> Estabilidad frio\n3 -> Transitorio calor\n4 -> Estabilidad calor"
              # "Para el primer ciclo, detectamos el flanco de Run Program\ny almacenamos el tiempo incial.\nPara el resto de ciclos, detectamos que haya habido un cambio\nde segmento y que el actual sea 4 (Cuando empieza a enfriar)."
              n372 = local write "Program running"(TRUE ("Program running")) -> ()
              n373 = Select(t=u16 50, s="Pausa", f="Segmento") -> (s? t:f=w563:u16)
              n374 = Select(t=u16 20, s="Test", f=w563) -> (s? t:f=w560:u16)
              n375 = case shown="4" w560 {
                tunnel: "Setpoint Frío" -> [w586 w597 _ _ _ _ _]
                tunnel: "Setpoint Corte Frío" -> [w583 w596 w627 _ _ _ _]
                frame 0, Default {
                  n376 = local write "Cam_Write_Set_Temp"(TRUE ("Enable_Temp_write")) -> ()
                  n377 = local write "Setpoint Peltiers"(w586) -> ()
                  n378 = local write "Cam_Temp_write"(w586) -> ()
                  n379 = local write "Cam_Hum_write"(0.0 ("Cam_Hum_write")) -> ()
                  n380 = local write "Cam_Write_Set_Hum"(TRUE ("Cam_Write_Set_Hum")) -> ()
                  n381 = local read "mean_T_valves"() -> (w584:dbl)
                  n382 = local read "Entrada digital Bitron"() -> (w581:bool)
                  n383 = local read "DO H2 LAB"() -> (w582:bool)
                  n384 = Less Or Equal?(x=w584, y=w583) -> (x <= y?=w585:bool)
                  n385 = And(x=w582, y=w581) -> (x .and. y?=w580:bool)
                  n386 = case shown="True" w580 {
                    frame False {
                    }
                    frame True {
                      n387 = Tick Count (ms)() -> (millisecond timer value=w590:u32)
                      n388 = local write "Timer 3 (Inicio Transitorio Calor)"(w590) -> ()
                      n389 = local write "Segmento"(u16 3 ("Segmento_temp")) -> ()
                    }
                  }
                  n390 = case shown="True" w585 {
                    frame False {
                    }
                    frame True {
                      n391 = local write "DO H2 LAB"(TRUE ("DO H2 LAB")) -> ()
                    }
                  }
                }
                frame 1 {
                  # "Segmento escalon frío"
                  # "(Luego -38)"
                  # "(para debuggar -5)"
                  # "(Ahora para debuggar ponemos T amb)"
                  # "Segmento -40"
                  n392 = local write "Cam_Write_Set_Temp"(TRUE ("Enable_Temp_write")) -> ()
                  n393 = local write "Setpoint Peltiers"(w597) -> ()
                  n394 = local write "Cam_Temp_write"(w597) -> ()
                  n395 = local write "Cam_Write_Set_Hum"(TRUE ("Cam_Write_Set_Hum")) -> ()
                  n396 = local write "Cam_Hum_write"(0.0 ("Cam_Hum_write")) -> ()
                  n397 = local read "mean_T_valves"() -> (w593:dbl)
                  n398 = Add(x=w596, y=2.0) -> (x+y=w594:dbl)
                  n399 = Less Or Equal?(x=w593, y=w594) -> (x <= y?=w601:bool)
                  n400 = case shown="True" w601 {
                    frame False {
                      n401 = local write "enable_PI"(FALSE ("Enable_PI")) -> ()
                    }
                    frame True {
                      n402 = Tick Count (ms)() -> (millisecond timer value=→"Timer 2 (Inicio Estabilidad Frio)":u32)
                      n403 = local write "Segmento"(u16 2 ("Segmento_temp")) -> ()
                    }
                  }
                }
                frame 2 {
                  # "90 min en ms"
                  # "15 min en ms"
                  # "100 min en ms"
                  # "Segmento estabilidad frío"
                  # "Ponemos un boton para debugar"
                  # "Esperar a lectura digital"
                  # "Activar salida digital"
                  n404 = local write "Setpoint Peltiers"(w627) -> ()
                  n405 = local write "Cam_Temp_write"(w627) -> ()
                  n406 = local write "Cam_Write_Set_Temp"(TRUE ("Cam_Write_Set_Temp")) -> ()
                  n407 = local write "Cam_Write_Set_Hum"(FALSE ("Cam_Write_Set_Hum")) -> ()
                  n408 = Tick Count (ms)() -> (millisecond timer value=w621:u32)
                  n409 = local read "Timer 2 (Inicio Estabilidad Frio)"() -> (w618:u32)
                  n410 = local read "Timer 1 (Inicio transitorio frio)"() -> (w620:u32)
                  n411 = Subtract(x=w621, y=w618) -> (x-y=w619:u32)
                  n412 = Subtract(x=w621, y=w620) -> (x-y=w622:u32)
                  n413 = local read "DO H2 LAB"() -> (w607:bool)
                  n414 = Multiply(x=u32 60000, y="Tiempo minimo de ciclo") -> (x*y=w613:u32)
                  n415 = Less?(x=w622, y=w613) -> (x < y?=w625:bool)
                  n416 = Multiply(x=u32 60000, y="Tiempò en estabilidad de Frío") -> (x*y=w617:u32)
                  n417 = Greater Or Equal?(x=w619, y=w617) -> (x >= y?=w624:bool)
                  n418 = And(x="Entrada digital Bitron", y=w607) -> (x .and. y?=w605:bool)
                  n419 = Multiply(x=u32 60000, y="Tiempo maximo de ciclo") -> (x*y=w609:u32)
                  n420 = Greater Or Equal?(x=w622, y=w609) -> (x >= y?=w623:bool)
                  n421 = And(x=w625, y=w624) -> (x .and. y?=w626:bool)
                  n422 = Or(x=w623, y=w626) -> (x .or. y?=w608:bool)
                  n423 = case shown="True" w605 {
                    frame False {
                    }
                    frame True {
                      n424 = Tick Count (ms)() -> (millisecond timer value=→"Timer 3 (Inicio Transitorio Calor)":u32)
                      n425 = local write "Segmento"(u16 3 ("Segmento_temp")) -> ()
                    }
                  }
                  n426 = case shown="True" w608 {
                    frame False {
                    }
                    frame True {
                      n427 = local write "DO H2 LAB"(TRUE ("DO H2 LAB")) -> ()
                    }
                  }
                }
                frame 3 {
                  # "Segmento rampa calor"
                  # "Rampa camara climatica"
                  # "Habilitamos rampa PI desde -40"
                  # "estaba a40_ Igual interesaría bajar la humedad a 10 %"
                  n428 = local write "Rampa_pelt"(TRUE ("Rampa_cam")) -> ()
                  n429 = local write "Rampa_cam"(TRUE ("Rampa_cam")) -> ()
                  n430 = local write "enable_PI"(TRUE ("Enable_PI")) -> ()
                  n431 = local write "Cam_Write_Set_Temp"(TRUE ("Enable_Temp_write")) -> ()
                  n432 = local write "Cam_Write_Set_Hum"(TRUE ("Cam_Write_Set_Hum")) -> ()
                  n433 = local write "Cam_Hum_write"(10.0 ("Cam_Hum_write")) -> ()
                  n434 = local read "Setpoint calor cam"() -> (w637:dbl)
                  n435 = local read "Cam_Temp_read"() -> (w634:dbl)
                  n436 = Subtract(x=w637, y=5.0) -> (x-y=w635:dbl)
                  n437 = Greater Or Equal?(x=w634, y=w635) -> (x >= y?=w633:bool)
                  n438 = case shown="True" w633 {
                    frame False {
                    }
                    frame True {
                      n439 = Tick Count (ms)() -> (millisecond timer value=→"Timer 4 (Inicio Estabilidad Calor)":u32)
                      n440 = local write "Segmento"(u16 4 ("Segmento_temp")) -> ()
                    }
                  }
                }
                frame 4 {
                  # "Segmento estabilidad calor"
                  # "Ponemos un boton para debugar"
                  # "Esperar a lectura digital"
                  n441 = local write "Cam_Write_Set_Hum"(FALSE ("Cam_Write_Set_Hum")) -> ()
                  n442 = local write "Cam_Write_Set_Temp"(FALSE ("Enable_Temp_write")) -> ()
                  n443 = local read "Entrada digital Bitron"() -> (w646:bool)
                  n444 = case shown="False" w646 {
                    frame False {
                      n445 = Tick Count (ms)() -> (millisecond timer value=→"Timer 1 (Inicio transitorio frio)":u32)
                      n446 = local write "DO H2 LAB"(FALSE ("DO H2 LAB")) -> ()
                      n447 = local write "Segmento"(u16 1 ("Segmento_temp")) -> ()
                    }
                    frame True {
                    }
                  }
                }
                frame 20 {
                  w661 = FALSE ("enable_PI")
                  n448 = local write "Rampa_pelt"(w661) -> ()
                  n449 = local write "Rampa_cam"(w661) -> ()
                  n450 = Index Array(array="Test PWM") -> (element #1=w659:u32, element #2=w658:u32, element #3=w657:u32, element #4=w656:u32, element #5=w655:u32, element #6=w654:u32, element #7=w653:u32, element #8=w652:u32)  [unwired: 8 in]
                  n451 = local write "PWM 8 (%)"(w652) -> ()
                  n452 = local write "PWM 6 (%)"(w654) -> ()
                  n453 = local write "PWM 7 (%)"(w653) -> ()
                  n454 = local write "PWM 5 (%)"(w655) -> ()
                  n455 = local write "PWM 4 (%)"(w656) -> ()
                  n456 = local write "PWM 1 (%)"(w659) -> ()
                  n457 = local write "PWM 2 (%)"(w658) -> ()
                  n458 = local write "PWM 3 (%)"(w657) -> ()
                }
                frame 50 {
                  n459 = local write "Cam_Write_Set_Temp"(FALSE ("Cam_Write_Set_Temp")) -> ()
                  n460 = case shown="True" "Pausa entrar" {
                    frame False {
                    }
                    frame True {
                      n461 = local read "Rampa_pelt"() -> (w666:bool)
                      n462 = local read "Cam_Temp_write"() -> (w673:dbl)
                      n463 = local read "enable_PI"() -> (w672:bool)
                      n464 = local read "enable_PI"() -> (w667:bool)
                      n465 = flat-sequence {
                        tunnel: w673 -> [w682]
                        tunnel: [w682] -> w675
                        tunnel: w672 -> [w678]
                        tunnel: [w678] -> w671
                        tunnel: [w677] -> w668
                        tunnel: w667 -> [w677]
                        tunnel: w666 -> [w676]
                        tunnel: [w676] -> w665
                        tunnel: w675 -> [w686]
                        tunnel: [w686] -> w674
                        tunnel: w671 -> [w685]
                        tunnel: [w685] -> w670
                        tunnel: [w684] -> w669
                        tunnel: w668 -> [w684]
                        tunnel: w665 -> [w683]
                        tunnel: [w683] -> w664
                        tunnel: w674 -> [w694]
                        tunnel: w670 -> [w692]
                        tunnel: w669 -> [w691]
                        tunnel: w664 -> [w690]
                        frame #0 {
                          w679 = FALSE ("Enable_PI")
                          n466 = local write "Cam_Write_Set_Temp"(TRUE ("Cam_Write_Set_Temp")) -> ()
                          n467 = local write "Cam_Temp_write"(25.0 ("Setpoint_temp_write")) -> ()
                          n468 = local write "Rampa_pelt"(w679) -> ()
                          n469 = local write "enable_PI"(w679) -> ()
                          n470 = local write "enable_PI"(w679) -> ()
                        }
                        frame #1 {
                          n471 = while {
                            stop <- w689 stop-if-true
                            n472 = local read "Pausa entrar"() -> (w688:bool)
                            n473 = Wait (ms)(milliseconds to wait=u32 200) -> ()  [unwired: 1 out]
                            n474 = Not(x=w688) -> (.not. x?=w689:bool)
                          }
                        }
                        frame #2 {
                          n475 = local write "Cam_Write_Set_Temp"(TRUE ("Cam_Write_Set_Temp")) -> ()
                          n476 = local write "Cam_Temp_write"(w694) -> ()
                          n477 = local write "Rampa_pelt"(w690) -> ()
                          n478 = local write "enable_PI"(w692) -> ()
                          n479 = local write "enable_PI"(w691) -> ()
                        }
                        frame #3 {
                          n480 = Wait (ms)(milliseconds to wait=u32 500) -> ()  [unwired: 1 out]
                        }
                      }
                    }
                  }
                }
              }
              n481 = local read "Test"() -> (w556:bool)
              n482 = case shown="False" w556 {
                frame False {
                  n483 = local write "Disable PID"(FALSE ("Disable PID")) -> ()
                  n484 = property on="Disable PID" class="Bool (strict)"("DisabledEnum"=T2."Disabled" ("Disabled")) -> ()  [unwired: 2 in, 2 out]
                }
                frame True {
                  n485 = property on="Disable PID" class="Bool (strict)"("DisabledEnum"=T2."Enabled" ("Disabled")) -> ()  [unwired: 2 in, 2 out]
                }
              }
              n486 = local read "STOP ALL"() -> (w567:bool)
              n487 = Or(x=w567, y="stop Control General") -> (x .or. y?=w558:bool)
              n488 = case shown="True" w558 {
                selector: w558 -> [_ w578]
                tunnel: [FALSE w578] -> w557
                frame False {
                }
                frame True {
                  w579 = u32 0 ("PWM 1 (%)")
                  n489 = local write "Disable PID"(FALSE ("Disable PID")) -> ()
                  n490 = local write "PWM 8 (%)"(w579) -> ()
                  n491 = local write "PWM 6 (%)"(w579) -> ()
                  n492 = local write "PWM 7 (%)"(w579) -> ()
                  n493 = local write "PWM 5 (%)"(w579) -> ()
                  n494 = local write "PWM 4 (%)"(w579) -> ()
                  n495 = local write "PWM 1 (%)"(w579) -> ()
                  n496 = local write "PWM 2 (%)"(w579) -> ()
                  n497 = local write "PWM 3 (%)"(w579) -> ()
                }
              }
              n498 = Wait (ms)(milliseconds to wait=u32 200) -> ()  [unwired: 1 out]
            }
            n499 = local write "Run Program"(w555) -> ()
          }
        }
        n500 = local read "STOP ALL"() -> (w550:bool)
        n501 = node-c288() -> ()  [unwired: 1 in, 1 out]
        "Program running" <- w549
        "First Time" <- TRUE
      }
      n502 = node-c288() -> (w52:T3)  [unwired: 4 in]
      n503 = timed-loop "Simulación señal Bitron" {
        timing: w40 -> [_]
        timing-out: [_] -> w39
        stop <- w492 stop-if-true
        w491 = 0 ("FSM Bitron Simulacion")
        n504 = node-c288() -> ()  [unwired: 1 in, 1 out]
        n505 = local read "Run Program"() -> (w490:bool)
        n506 = And(x=w490, y="Activar Sim Bitron") -> (x .and. y?=w489:bool)
        n507 = case shown="False" w489 {
          tunnel: w491 -> [_ _]
          frame False {
          }
          frame True {
            n508 = disable-structure shown="Enabled" {
              frame Disabled {
                n509 = flat-sequence {
                  tunnel: [w502] -> w495
                  tunnel: w495 -> [w519]
                  frame #0 {
                    (unwired) 90.0 ("y")
                    w510 = u64 0 ("t")
                    n510 = First Call?() -> (First Call?: T/F=w515:bool)
                    n511 = case shown="True" w515 {
                      frame False {
                      }
                      frame True {
                        n512 = local write "Entrada digital Bitron"(FALSE ("Entrada digital Bitron")) -> ()
                      }
                    }
                    n513 = feedback #6(w510) -> (w508:u64)
                    n514 = Select(t=w510, s="Reset tempo", f=w508) -> (s? t:f=w497:u64)
                    "t ensayo (s)" <- w497
                    n515 = Increment(x=w497) -> (x+1=w509:u64)
                    n516 = feedback-in #6(w509) -> ()
                    n517 = To Double Precision Float(number=w497) -> (double precision float=w511:dbl)
                    n518 = Quotient & Remainder(x=w511, y=60.0) -> (x-y*floor(x/y)=→"segundos":dbl, floor(x/y)=w506:dbl)
                    "Minutos Totales" <- w506
                    n519 = Quotient & Remainder(x=w506, y="Minutos de medio ciclo") -> (floor(x/y)=w502:dbl)  [unwired: 1 out]
                    n520 = Quotient & Remainder(x=w506, y=60.0) -> (x-y*floor(x/y)=→"Minutos":dbl, floor(x/y)=w505:dbl)
                    n521 = Divide(x=w502, y=2.0) -> (x/y=→"Ciclos Totales":dbl)
                    n522 = Quotient & Remainder(x=w505, y=24.0) -> (x-y*floor(x/y)=→"Horas":dbl, floor(x/y)=→"días":dbl)
                  }
                  frame #1 {
                    n523 = feedback-in #7(w519) -> ()
                    n524 = feedback #7(w519) -> (w518:dbl)
                    n525 = Not Equal?(x=w519, y=w518) -> (x != y?=w517:bool)
                    n526 = case shown="True" w517 {
                      frame False {
                      }
                      frame True {
                        n527 = local read "Entrada digital Bitron"() -> (w520:bool)
                        n528 = Not(x=w520) -> (.not. x?=w521:bool)
                        n529 = local write "Entrada digital Bitron"(w521) -> ()
                      }
                    }
                  }
                }
              }
              frame Enabled {
                n530 = while {
                  stop <- w522 stop-if-true
                  n531 = Wait (ms)(milliseconds to wait=u32 500) -> ()  [unwired: 1 out]
                  n532 = local read "stop Control General"() -> (w524:bool)
                  n533 = local read "STOP ALL"() -> (w523:bool)
                  n534 = case shown="1" "FSM Bitron Simulacion" {
                    frame 1 {
                      n535 = flat-sequence {
                        frame #0 {
                          n536 = Tick Count (ms)() -> (millisecond timer value=w527:u32)
                          n537 = while {
                            tunnel: w527 -> [w537]
                            stop <- w531 stop-if-true
                            # "70 min  de ciclo"
                            n538 = Tick Count (ms)() -> (millisecond timer value=w538:u32)
                            n539 = Wait (ms)(milliseconds to wait=u32 500) -> ()  [unwired: 1 out]
                            n540 = Subtract(x=w538, y=w537) -> (x-y=w530:u32)
                            n541 = local read "stop Control General"() -> (w534:bool)
                            n542 = local read "STOP ALL"() -> (w535:bool)
                            n543 = Multiply(x=u32 60000 ("milliseconds to wait"), y="T cliclo (Bitron FSM Sim)") -> (x*y=w529:u32)
                            n544 = Greater Or Equal?(x=w530, y=w529) -> (x >= y?=w532:bool)
                            n545 = Or(x=w535, y=w534) -> (x .or. y?=w533:bool)
                            n546 = Or(x=w532, y=w533) -> (x .or. y?=w531:bool)
                          }
                        }
                        frame #1 {
                          n547 = local write "FSM Bitron Simulacion"(0 ("FSM Bitron Simulacion")) -> ()
                          n548 = local write "Entrada digital Bitron"(FALSE ("Entrada digital Bitron")) -> ()
                        }
                      }
                    }
                    frame 0, Default {
                      n549 = local read "DO H2 LAB"() -> (w542:bool)
                      n550 = case shown="True" w542 {
                        frame False {
                        }
                        frame True {
                          n551 = local write "FSM Bitron Simulacion"(1 ("FSM Bitron Simulacion")) -> ()
                          n552 = local write "Entrada digital Bitron"(TRUE ("Entrada digital Bitron")) -> ()
                        }
                      }
                    }
                  }
                  n553 = Or(x=w523, y=w524) -> (x .or. y?=w522:bool)
                }
              }
            }
          }
        }
        n554 = local write "FSM Bitron Simulacion"(w491) -> ()
        n555 = local read "STOP ALL"() -> (w492:bool)
        n556 = node-c288() -> ()  [unwired: 1 in, 1 out]
      }
      n557 = node-c288() -> (w54:T3)  [unwired: 4 in]
      n558 = timed-loop "Modbus Camara climatica" {
        timing: w52 -> [_]
        timing-out: [_] -> w51
        shift-right: [w712] -> w47
        shift-left: w50 -> [w716]
        shift-right: [w711] -> w48
        shift-left: w49 -> [w715]
        stop <- w700 stop-if-true
        n559 = node-c288() -> (→"Iteration Duration":i64)  [unwired: 1 in, 1 out]
        n560 = call "Eurotherm_read_TH.vi"("Modbus Master in"=w716, "error in (no error)"=w715) -> ("HR_rd"=w704:dbl, "Modbus Master out"=w714:refnum<class "Modbus Master.lvclass">, "Tª_rd"=→"Cam_Temp_read":dbl, "error out"=w713:errorcluster)  [unwired: 14 in]
        "Cam_Hum_read" <- w704
        n561 = local read "STOP ALL"() -> (w701:bool)
        n562 = Select(t=w704, s="Desconex_Control_Hum", f="Cam_Hum_write") -> (s? t:f=w706:dbl)
        n563 = case shown="False" w701 {
          selector: w701 -> [w717 w728]
          tunnel: w714 -> [w727 w738]
          tunnel: w713 -> [w723 w737]
          tunnel: [w725 w734] -> w712
          tunnel: [w724 w733] -> w711
          tunnel: "Cam_Write_Set_Temp" -> [_ w732]
          tunnel: "Cam_Temp_write" -> [_ w731]
          tunnel: "Cam_Write_Set_Hum" -> [_ w730]
          tunnel: w706 -> [_ w729]
          tunnel: [w717 w728] -> w700
          frame True {
            n564 = call "Eurotherm_write_T.vi"("error in (no error)"=w723, "Tª_sp"=25.0, "Tª write"=TRUE, "Modbus Master in"=w727) -> ("error out"=w722:errorcluster, "Modbus Master out"=w726:refnum<class "Modbus Master.lvclass">)  [unwired: 6 in]
            n565 = call "Eurotherm_write_H.vi"("error in (no error)"=w722, "HR_sp"=40.0, "HR write"=TRUE, "Modbus Master in"=w726) -> ("error out"=w724:errorcluster, "Modbus Master out"=w725:refnum<class "Modbus Master.lvclass">)  [unwired: 6 in]
          }
          frame False {
            n566 = call "Eurotherm_write_T.vi"("error in (no error)"=w737, "Tª_sp"=w731, "Tª write"=w732, "Modbus Master in"=w738) -> ("error out"=w735:errorcluster, "Modbus Master out"=w736:refnum<class "Modbus Master.lvclass">)  [unwired: 6 in]
            n567 = call "Eurotherm_write_H.vi"("error in (no error)"=w735, "HR_sp"=w729, "HR write"=w730, "Modbus Master in"=w736) -> ("error out"=w733:errorcluster, "Modbus Master out"=w734:refnum<class "Modbus Master.lvclass">)  [unwired: 6 in]
          }
        }
        n568 = node-c288() -> ()  [unwired: 1 in, 1 out]
      }
      n569 = timed-loop "Control Peltiers" {
        timing: w54 -> [_]
        timing-out: [_] -> w53
        stop <- w745 stop-if-true
        n570 = node-c288() -> ()  [unwired: 1 in, 1 out]
        n571 = case shown="False" "Disable PID" {
          frame True {
          }
          frame False {
            n572 = local read "T_valves"() -> (w755:dbl[])
            n573 = Index Array(array=w755, index #1=0 ("index")) -> (element #1=w753:dbl, element #2=w752:dbl, element #3=w751:dbl, element #4=w750:dbl, element #5=w749:dbl, element #6=w748:dbl, element #7=w747:dbl, element #8=w746:dbl)  [unwired: 7 in]
            n574 = call "PI_valvulas.vi"("controlON"="enable_PI", "Temperatura"=w753, "Setpoint T"="Setpoint Peltiers") -> ("PWM (%)"=w770:dbl)  [unwired: 8 in]
            n575 = call "PI_valvula5.vi"("controlON"="enable_PI", "Temperatura"=w749, "Setpoint T"="Setpoint Peltiers") -> ("PWM (%)"=w759:dbl)  [unwired: 8 in]
            n576 = To Unsigned Long Integer(number=w770) -> (unsigned 32bit integer=→"PWM 1 (%)":u32)
            n577 = To Unsigned Long Integer(number=w759) -> (unsigned 32bit integer=→"PWM 5 (%)":u32)
            n578 = call "PI_valvula2.vi"("controlON"="enable_PI", "Temperatura"=w752, "Setpoint T"="Setpoint Peltiers") -> ("PWM (%)"=w773:dbl)  [unwired: 8 in]
            n579 = call "PI_valvula6.vi"("controlON"="enable_PI", "Temperatura"=w748, "Setpoint T"="Setpoint Peltiers") -> ("PWM (%)"=w758:dbl)  [unwired: 8 in]
            n580 = To Unsigned Long Integer(number=w758) -> (unsigned 32bit integer=→"PWM 6 (%)":u32)
            n581 = To Unsigned Long Integer(number=w773) -> (unsigned 32bit integer=→"PWM 2 (%)":u32)
            n582 = call "PI_valvula7.vi"("controlON"="enable_PI", "Temperatura"=w747, "Setpoint T"="Setpoint Peltiers") -> ("PWM (%)"=w757:dbl)  [unwired: 8 in]
            n583 = call "PI_valvula3.vi"("controlON"="enable_PI", "Temperatura"=w751, "Setpoint T"="Setpoint Peltiers") -> ("PWM (%)"=w766:dbl)  [unwired: 8 in]
            n584 = To Unsigned Long Integer(number=w766) -> (unsigned 32bit integer=→"PWM 3 (%)":u32)
            n585 = To Unsigned Long Integer(number=w757) -> (unsigned 32bit integer=→"PWM 7 (%)":u32)
            n586 = call "PI_valvula8.vi"("controlON"="enable_PI", "Temperatura"=w746, "Setpoint T"="Setpoint Peltiers") -> ("PWM (%)"=w756:dbl)  [unwired: 8 in]
            n587 = call "PI_valvula4.vi"("controlON"="enable_PI", "Temperatura"=w750, "Setpoint T"="Setpoint Peltiers") -> ("PWM (%)"=w767:dbl)  [unwired: 8 in]
            n588 = To Unsigned Long Integer(number=w756) -> (unsigned 32bit integer=→"PWM 8 (%)":u32)
            n589 = To Unsigned Long Integer(number=w767) -> (unsigned 32bit integer=→"PWM 4 (%)":u32)
          }
        }
        n590 = local read "STOP ALL"() -> (w745:bool)
        n591 = node-c288() -> ()  [unwired: 1 in, 1 out]
      }
      n592 = node-c288(w51) -> ()  [unwired: 1 out]
      n593 = node-c288(w53) -> ()  [unwired: 1 out]
      n594 = node-c288(w39) -> ()  [unwired: 1 out]
      n595 = node-c288(w45) -> ()  [unwired: 1 out]
    }
    frame #2 {
      w811 = u32 0 ("PWM_DO0")
      # "End"
      n596 = call-dynamic "Close.vi"("error in (no error)"=w809, "Modbus master in"=w810) -> ("error out"=w808:errorcluster)  [unwired: 9 in]
      n597 = call-dynamic "Close.vi"("error in (no error)"=w823, "Modbus master in"=w822) -> ("error out"=w820:errorcluster)  [unwired: 9 in]
      n598 = local write "STOP ALL"(FALSE ("stop")) -> ()
      n599 = local write "PWM 8 (%)"(w811) -> ()
      n600 = local write "PWM 6 (%)"(w811) -> ()
      n601 = local write "PWM 7 (%)"(w811) -> ()
      n602 = local write "PWM 5 (%)"(w811) -> ()
      n603 = local write "PWM 4 (%)"(w811) -> ()
      n604 = local write "PWM 1 (%)"(w811) -> ()
      n605 = local write "PWM 2 (%)"(w811) -> ()
      n606 = xnode "Read/Write Control"("FPGA VI Reference In"=w815, "error in"=w814) -> ("FPGA VI Reference Out"=w813:refnum<k20>, "error out"=w812:errorcluster)  [unwired: 8 in]
      n607 = local write "PWM 3 (%)"(w811) -> ()
      n608 = call <vilib>:"DAQmx Stop Task.vi"("task/channels in"=w818, "error in"=w817) -> ("error out"=w816:errorcluster)  [unwired: 12 in, 1 out]
      n609 = xnode "Close FPGA VI Reference"("FPGA VI Reference In"=w813, "error in"=w812) -> ("error out"=w819:errorcluster)
      n610 = Merge Errors(w816, w819, w820, w808) -> (w821:errorcluster)
      n611 = call <vilib>:"Simple Error Handler.vi"("error in (no error)"=w821) -> ()  [unwired: 4 in, 5 out]
    }
  }
